vi "Run.vi"(8 "error in (no error)":errorcluster, 9 "s on last turn":dbl=0.3439976484514773, 10 "Maze (0: Empty, -1: Enemy. >0: Teammate":i32[][](array[numeric])=[[16, 0, 18], [0, 14, 0], [0, 0, 0]], 11 "Mother In":refnum<class "Formics.lvclass">=refnum) -> (0 "error out":errorcluster, 1 "Direction":T1=enum."SE", 2 "Action":T2=enum."Replicate", 3 "Mother Out":refnum<class "Formics.lvclass">, 4 "Replicated":refnum<class "Square.lvclass">)   [LabVIEW 2015, in "Formics.lvclass"]
uses:
  Formics.lvclass
  Type Defs/Action Enum.ctl
  Type Defs/Direction Enum.ctl
  Square/Square.lvclass
  Formics.lvclass/Formics.ctl
  Attack Options.ctl
  Common/Common.lvlib
  Type Defs/SB Type Defs.lvlib
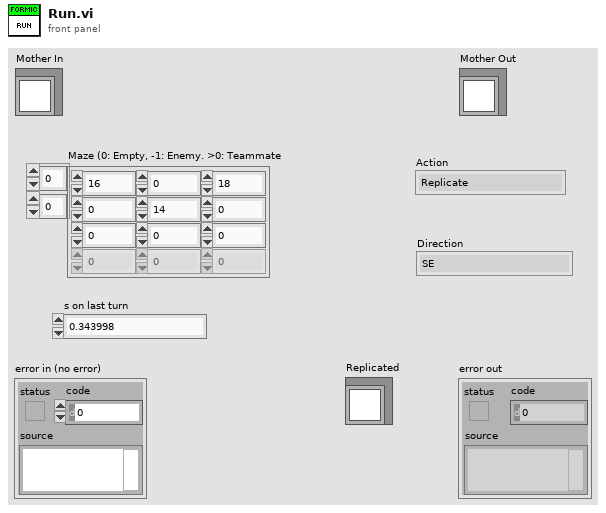
[diagram p1: front panel]
types:
  T1 = typedef "SB Type Defs.lvlib/Direction Enum.ctl" = enum16{"NW", "N", "NE", "E", "SE", "S", "SW", "W"}
  T2 = typedef "SB Type Defs.lvlib/Action Enum.ctl" = enum16{"Wait", "Move", "Attack", "Replicate"}
  T3 = typedef "Formics.lvclass/Kamikaze DVR.ctl" = refnum<data-value>
  T4 = typedef "Formics.lvclass/Current Directive.ctl" = enum16{"Queen", "Daughter", "Coward", "Migrate", "Line Up", "Protector", "Scout"}
  T5 = typedef "Formics.lvclass/Attack Options.ctl" = enum16{"Attack", "Run", "Distract"}
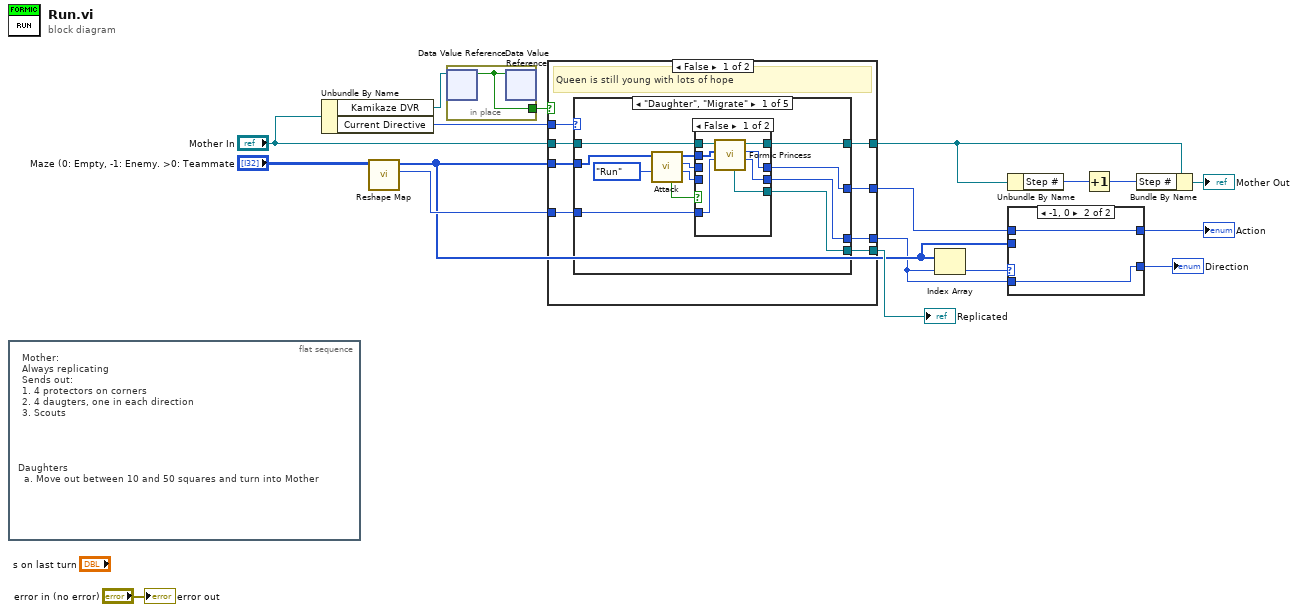
[diagram p0: block diagram]
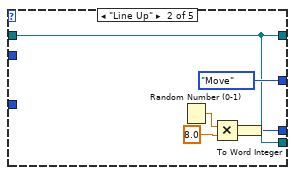
[diagram p3: hidden frame]
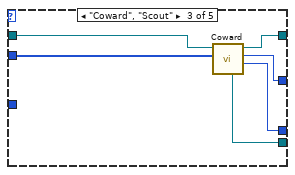
[diagram p4: hidden frame]
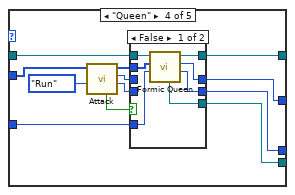
[diagram p5: hidden frame]
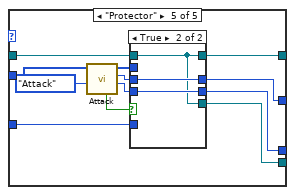
[diagram p7: hidden frame]
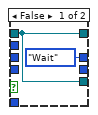
[diagram p8: hidden frame]
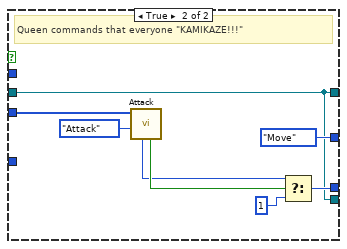
[diagram p9: hidden frame]
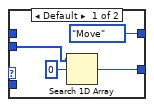
[diagram p10: hidden frame]
diagram:
  n1 = flat-sequence {
    frame #0 {
      # "Daughters\n  a. Move out between 10 and 50 squares and turn into Mother"
      # "Mother:\nAlways replicating\nSends out:\n1. 4 protectors on corners\n2. 4 daugters, one in each direction\n3. Scouts"
    }
  }
  n2 = Unbundle By Name("Mother In") -> ("Kamikaze DVR"=w6:T3, "Current Directive"=w13:T4)
  n3 = call "Reshape Map.vi"("Maze (0: Empty, -1: Enemy. >0: Teammate"="Maze (0: Empty, -1: Enemy. >0: Teammate") -> ("SelfID"=w14:i32, "Map"=w3:i32[])  [unwired: 9 in]
  n4 = in-place {
    in-place-border: [w19] -> w5
    n5 = in-place-dvr #1(w6) -> (w19:bool)  [unwired: 1 out]
    n6 = in-place-dvr #1(w19) -> ()  [unwired: 2 out]
  }
  n7 = case shown="False" w5 {
    tunnel: w3 -> [w27 w107]
    tunnel: w14 -> [w26 _]
    tunnel: w13 -> [w25 _]
    tunnel: "Mother In" -> [w24 w101]
    tunnel: [w23 w104] -> w1
    tunnel: [w22 w101] -> w11
    tunnel: [w21 w101] -> w4
    tunnel: [w20 Action_Enum."Move" ("Action")] -> w10
    frame False {
      # "Queen is still young with lots of hope"
      n8 = case shown="\"Daughter\", \"Migrate\"" w25 {
        tunnel: w24 -> [w39 w52 w61 w73 w95]
        tunnel: [w38 w52 w60 w72 w94] -> w22
        tunnel: w27 -> [w37 _ w56 w70 w92]
        tunnel: w26 -> [w32 _ _ w68 w90]
        tunnel: [w28 w50 w58 w63 w85] -> w23
        tunnel: [w34 w52 w57 w66 w88] -> w21
        tunnel: [w33 Action_Enum."Move" ("Action") w59 w67 w89] -> w20
        frame "Daughter", "Migrate" {
          n9 = call "Attack.vi"("Attack?"=Attack_Options."Run", "Maze (0: Empty, -1: Enemy. >0: Teammate"=w37) -> ("Direction"=w29:i32, "Action"=w30:T2, "Maze (0: Empty, -1: Enemy. >0: Teammate 2"=w36:i32[], "Enemy Found?"=w31:bool)  [unwired: 4 in, 2 out]
          n10 = case shown="False" w31 {
            tunnel: w39 -> [w46 w49]
            tunnel: [w45 w49] -> w38
            tunnel: w36 -> [w44 _]
            tunnel: [w43 w49] -> w34
            tunnel: [w42 w48] -> w33
            tunnel: w32 -> [w41 _]
            tunnel: w30 -> [_ w48]
            tunnel: w29 -> [_ w47]
            tunnel: [w40 w47] -> w28
            frame False {
              n11 = call "Formic Princess.vi"("SelfID"=w41, "Map"=w44, "Mother in"=w46) -> ("Direction"=w40:T1, "Action"=w42:T2, "Mother out"=w45:refnum<class "Formics.lvclass">, "Replicated Class"=w43:refnum<class "Formics.lvclass">)  [unwired: 4 in, 1 out]
            }
            frame True {
            }
          }
        }
        frame "Line Up" {
          n12 = Random Number (0-1)() -> (number: 0 to 1=w54:dbl)
          n13 = Multiply(x=w54, y=8.0) -> (x*y=w51:dbl)
          n14 = To Word Integer(number=w51) -> (16bit integer=w50:i16)
        }
        frame "Coward", "Scout" {
          n15 = call-dynamic "Coward.vi"("Map"=w56, "Mother In"=w61) -> ("Direction"=w58:T1, "Action"=w59:T2, "Mother Out"=w60:refnum<class "Formics.lvclass">, "Replicated"=w57:refnum<class "Square.lvclass">)  [unwired: 5 in, 1 out]
        }
        frame "Queen" {
          n16 = call "Attack.vi"("Attack?"=Attack_Options."Run", "Maze (0: Empty, -1: Enemy. >0: Teammate"=w70) -> ("Direction"=w64:i32, "Action"=w65:T2, "Maze (0: Empty, -1: Enemy. >0: Teammate 2"=w69:i32[], "Enemy Found?"=w62:bool)  [unwired: 4 in, 2 out]
          n17 = case shown="False" w62 {
            tunnel: w73 -> [w80 w81]
            tunnel: [w79 w81] -> w72
            tunnel: w69 -> [w78 _]
            tunnel: w68 -> [w77 _]
            tunnel: [w76 w83] -> w67
            tunnel: [w75 w81] -> w66
            tunnel: w65 -> [_ w83]
            tunnel: w64 -> [_ w82]
            tunnel: [w74 w82] -> w63
            frame False {
              n18 = call "Formic Queen.vi"("SelfID"=w77, "Map"=w78, "Mother in"=w80) -> ("Direction"=w74:T1, "Action"=w76:T2, "Mother out"=w79:refnum<class "Formics.lvclass">, "Replicated Class"=w75:refnum<class "Formics.lvclass">)  [unwired: 4 in, 1 out]
            }
            frame True {
            }
          }
        }
        frame "Protector" {
          n19 = call "Attack.vi"("Attack?"=Attack_Options."Attack", "Maze (0: Empty, -1: Enemy. >0: Teammate"=w92) -> ("Direction"=w86:i32, "Action"=w87:T2, "Maze (0: Empty, -1: Enemy. >0: Teammate 2"=w91:i32[], "Enemy Found?"=w84:bool)  [unwired: 4 in, 2 out]
          n20 = case shown="True" w84 {
            tunnel: w95 -> [w97 w98]
            tunnel: [w97 w98] -> w94
            tunnel: w91 -> [_ _]
            tunnel: w90 -> [_ _]
            tunnel: [Action_Enum."Wait" ("Action") w100] -> w89
            tunnel: [w97 w98] -> w88
            tunnel: w87 -> [_ w100]
            tunnel: w86 -> [_ w99]
            tunnel: [_ w99] -> w85
            frame False {
            }
            frame True {
            }
          }
        }
      }
    }
    frame True {
      # "Queen commands that everyone \"KAMIKAZE!!!\""
      n21 = call "Attack.vi"("Attack?"=Attack_Options."Attack", "Maze (0: Empty, -1: Enemy. >0: Teammate"=w107) -> ("Enemy Found?"=w106:bool, "Enemy Direction"=w105:i32)  [unwired: 4 in, 4 out]
      n22 = Select(t=w105, s=w106, f=1) -> (s? t:f=w104:i32)
    }
  }
  "Replicated" <- w4
  n23 = Index Array(array=w3, index=w1) -> (element=w17:i32)
  n24 = Unbundle By Name(w11) -> ("Step #"=w8:i32)
  n25 = case shown="-1, 0" w17 {
    tunnel: w10 -> [_ w114]
    tunnel: [Action_Enum."Move" ("Action") w114] -> w16
    tunnel: w3 -> [w111 _]
    tunnel: [w109 w113] -> w2
    tunnel: w1 -> [_ w113]
    frame Default {
      n26 = Search 1D Array(1D array=w111, element=0) -> (index of element=w109:i32)  [unwired: 1 in]
    }
    frame -1, 0 {
    }
  }
  "Action" <- w16
  "Direction" <- w2
  n27 = Increment(x=w8) -> (x+1=w7:i32)
  n28 = Bundle By Name(cluster=w11, "Step #"=w7) -> (→"Mother Out":refnum<class "Formics.lvclass">)
  "error out" <- "error in (no error)"
